vi "coerce_to_range.vi"(0 "error in (no error) 2":errorcluster, 3 "channel no.":u8, 4 "x":u8, 5 "lower limit":u8, 6 "upper limit":u8) -> (1 "coerced(x)":u8, 2 "error in (no error)":errorcluster)   [LabVIEW 2021]
panel:
  out "In Range?":bool
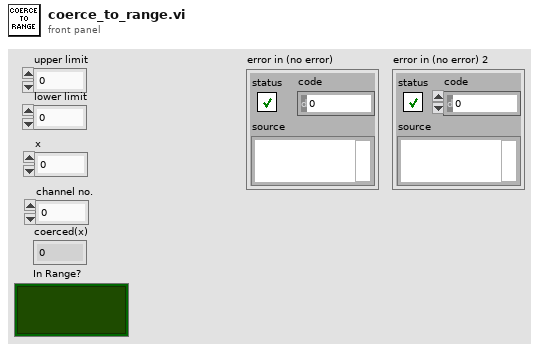
[diagram p1: front panel]
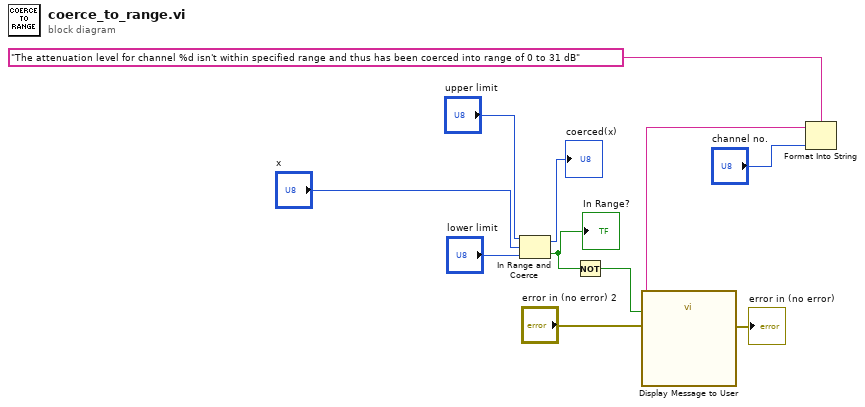
[diagram p0: block diagram]
diagram:
  n1 = In Range and Coerce(upper limit="upper limit", x="x", lower limit="lower limit") -> (coerced(x)=→"coerced(x)":u8, In Range?=w5:bool)
  "In Range?" <- w5
  n2 = Not(x=w5) -> (.not. x?=w4:bool)
  n3 = Format Into String(format string="The attenuation level for channel %d isn't within specified range and thus has been coerced into range of 0 to 31 dB" ("Message"), "channel no.") -> (resulting string=w1:string)  [unwired: 2 in, 1 out]
  n4 = call "Display Message to User"("error in (no error)"="error in (no error) 2", "Enable"=w4, "Message"=w1) -> ("error out"=→"error in (no error)":errorcluster)  [unwired: 7 in, 1 out]
